vi "AutoWriterContainer.vi"(0 "Mode(Write=True)":bool, 2 "Input":i16[](array[numeric])=[0]) -> (1 "Output":i16[](array[numeric]))   [LabVIEW 2010, in "Recorder.lvlib"]
uses:
  Recorder.lvlib
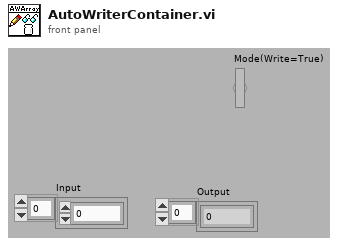
[diagram p1: front panel]
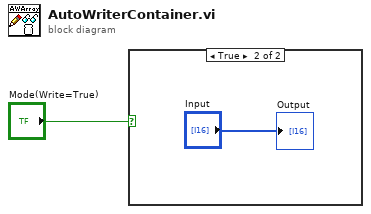
[diagram p0: block diagram]
diagram:
  n1 = case shown="True" "Mode(Write=True)" {
    frame False {
    }
    frame True {
      "Output" <- "Input"
    }
  }
